vi "Start Triggers Sync AUX Core.vi"(0 "sync.resources":T2, 1 "rx 0.stream enable":bool, 2 "rx 1.stream enable":bool, 3 "tx 0.stream enable":bool, 4 "tx 1.stream enable":bool, 6 "rx.trigger select":T1=enum."Immediate", 7 "tx.trigger select":T1=enum."Immediate", 8 "rx.software trigger":bool, 9 "tx.software trigger":bool, 10 "rx.trigger enable":bool, 11 "tx.trigger enable":bool, 12 "rx.trigger sync enable":bool, 13 "tx.trigger sync enable":bool) -> (14 "rx.start trigger":bool, 15 "tx.start trigger":bool)   [LabVIEW 2023]
uses:
  <instrlib>/niUSRPRIO/Synchronization/v1/FPGA/niUsrpRio Synchronization v1 FPGA.lvlib
  <instrlib>/niUSRPRIO/Synchronization/v1/FPGA/Private/Resources.ctl
  <instrlib>/niVST/Reference FPGA/FPGA/USRPRIO Sample VIs/Host/SubVIs/Start Trigger.ctl
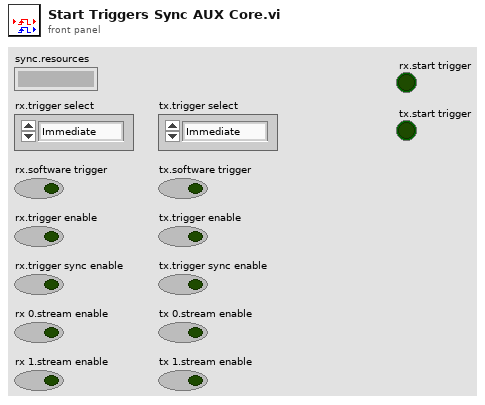
[diagram p1: front panel]
types:
  T1 = typedef "Start Trigger.ctl" = enum8{"Software", "Digital Edge", "Rx Start Trigger", "Tx Start Trigger", "Immediate", "Future Time Event"}
  T2 = typedef "niUsrpRio Synchronization v1 FPGA.lvlib/Resources.ctl" = cluster{"master":refnum<k21>, "meas.enable":refnum<k21>, "meas.ready":refnum<k21>, "meas.reset":refnum<k21>, "meas.arm":refnum<k21>, "meas.valid":refnum<k21>, "meas.value":refnum<k21>, "meas.oversample factor":refnum<k21>, "cptr":refnum<k21>, "cptr.adjust":refnum<k21>, "cptr.period":refnum<k21>}
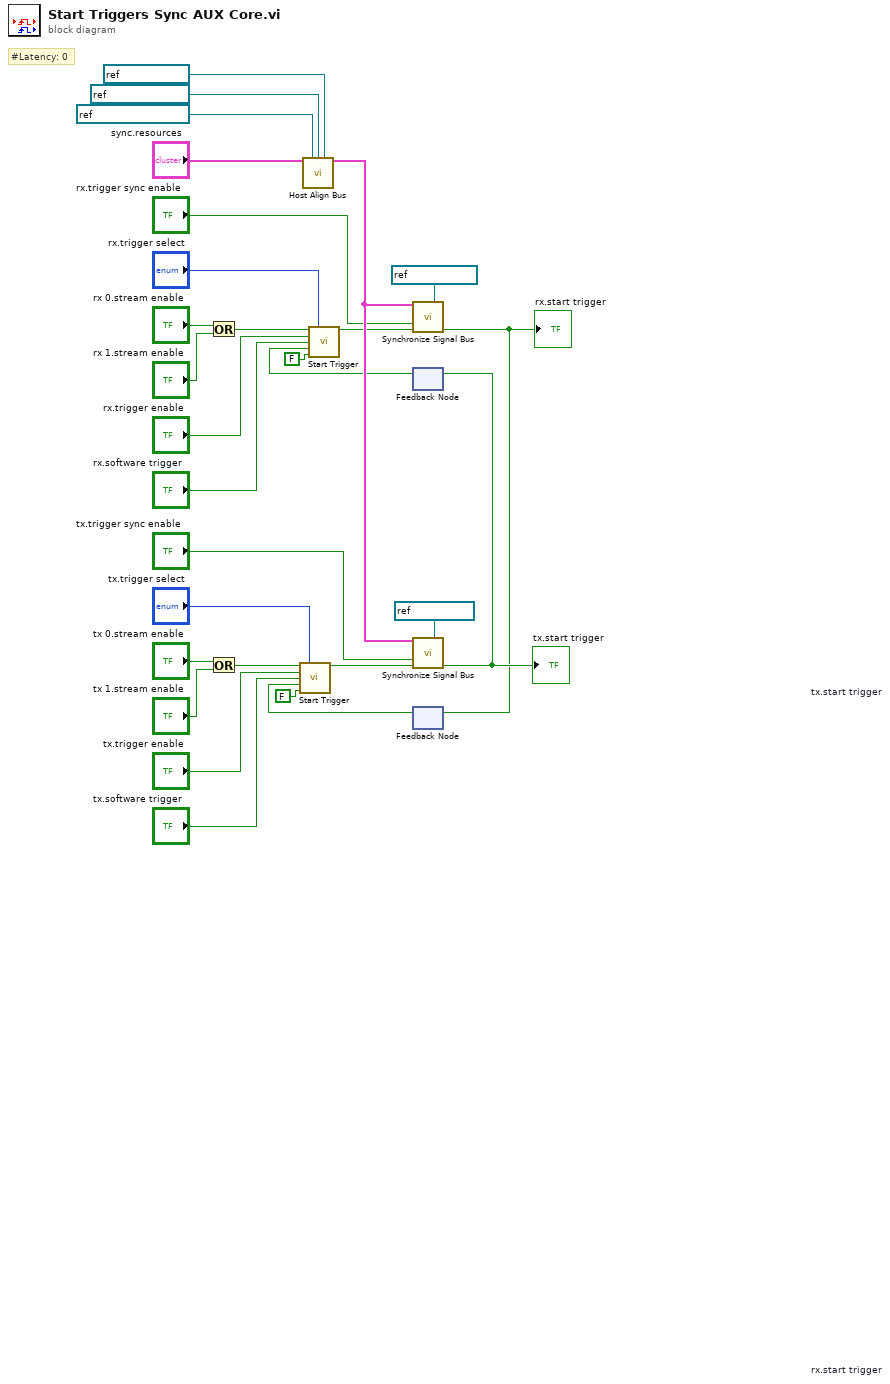
[diagram p0: block diagram]
diagram:
  # "#Latency: 0"
  n1 = Or(x="rx 0.stream enable", y="rx 1.stream enable") -> (x .or. y?=w16:bool)
  n2 = Or(x="tx 0.stream enable", y="tx 1.stream enable") -> (x .or. y?=w12:bool)
  n3 = call <instrlib>:"Host Align Bus.vi"("sync.resources"="sync.resources", "common reference"=refnum<k21> "Reference Clock", "clock x2"=refnum<k21> "Data Clock x2", "sync.meas.fpga io"=refnum<k21> "AUX I/O 11") -> ("sync.resources"=w29:T2)  [unwired: 11 in]
  n4 = feedback #1 "tx.start trigger"() -> (w13:bool)  [unwired: 1 in]
  n5 = call <instrlib>:"Start Trigger.vi"("stream enable"=w16, "trigger select"="rx.trigger select", "trigger enable"="rx.trigger enable", "software trigger"="rx.software trigger", "other start trigger"=w13, "event occurred"=FALSE) -> ("start trigger"=w2:bool)  [unwired: 9 in]
  n6 = call <instrlib>:"Synchronize Signal Bus.vi"("sync.resources"=w29, "sync.fpga io"=refnum<k21> "AUX I/O 10", "enable"="rx.trigger sync enable", "edge"=w2) -> ("synchronized edge"=w1:bool)  [unwired: 9 in, 2 out]
  "rx.start trigger" <- w1
  n7 = feedback-in #2(w1) -> ()
  n8 = feedback #2 "rx.start trigger"() -> (w9:bool)  [unwired: 1 in]
  n9 = call <instrlib>:"Start Trigger.vi"("stream enable"=w12, "trigger select"="tx.trigger select", "trigger enable"="tx.trigger enable", "software trigger"="tx.software trigger", "other start trigger"=w9, "event occurred"=FALSE) -> ("start trigger"=w8:bool)  [unwired: 9 in]
  n10 = call <instrlib>:"Synchronize Signal Bus.vi"("sync.resources"=w29, "sync.fpga io"=refnum<k21> "AUX I/O 9", "enable"="tx.trigger sync enable", "edge"=w8) -> ("synchronized edge"=w7:bool)  [unwired: 9 in, 2 out]
  "tx.start trigger" <- w7
  n11 = feedback-in #1(w7) -> ()
